vi "Save.vi"() -> ()   [LabVIEW 2018]
uses:
  <vilib>/express/express shared/transition.llb/Dynamic To Waveform Array.vi
  <vilib>/express/express signal manip/GetorSetDDTAttributes/Set DDT Attributes/SetT0.vi
  <vilib>/express/express shared/transition.llb/Waveform Array To Dynamic.vi
  <vilib>/express/express signal manip/GetorSetDDTAttributes/Set DDT Attributes/Set DDT Properties.xnode
panel:
  in  "Stop":bool
  in  "Array":dbl[](array[numeric])
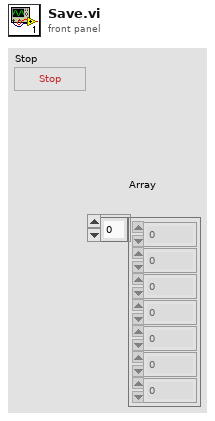
[diagram p1: front panel]
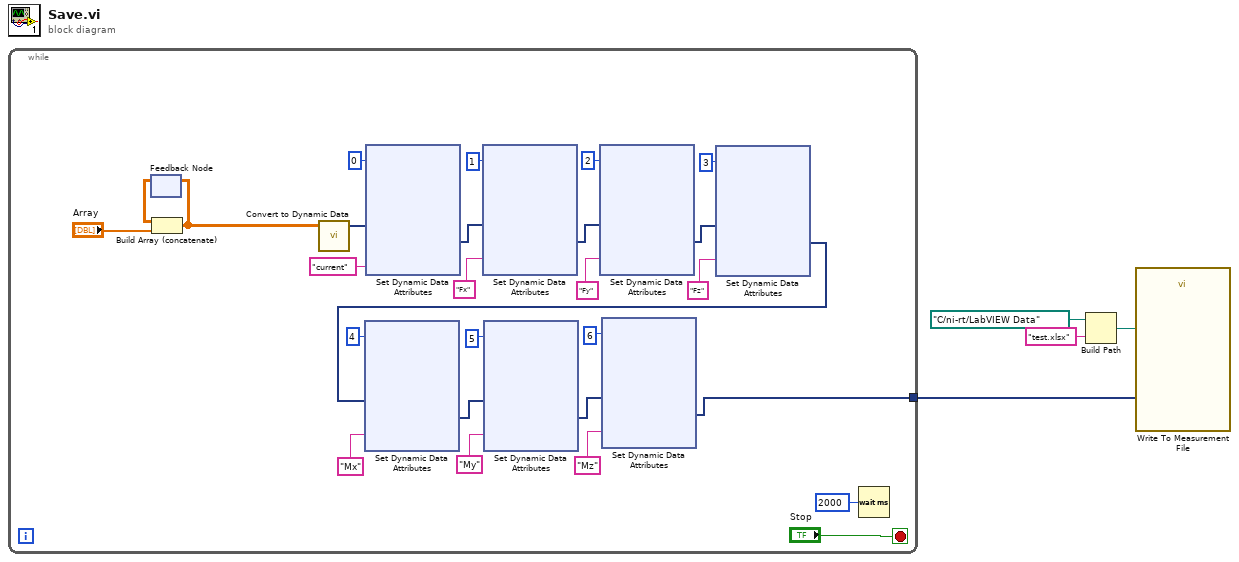
[diagram p0: block diagram]
diagram:
  n1 = while {
    tunnel: [w7] -> w1
    stop <- "Stop" stop-if-true
    n2 = feedback #1() -> (w10:dbl[][])  [unwired: 1 in]
    n3 = Build Array (concatenate)(w10, "Array") -> (w5:dbl[][])
    n4 = feedback-in #1(w5) -> ()
    n5 = call "Convert to Dynamic Data"("2D Array"=w5) -> ("Dynamic Data Type"=w30:dynamicdata)  [unwired: 3 in]
    n6 = xnode "Set Dynamic Data Attributes"("Signals In"=w30, "Signal Name"="current", "Signal Index"=0) -> ("Signals Out"=w28:dynamicdata)  [unwired: 1 in, 1 out]
    n7 = xnode "Set Dynamic Data Attributes"("Signals In"=w28, "Signal Name"="Fx", "Signal Index"=1) -> ("Signals Out"=w23:dynamicdata)  [unwired: 1 in, 1 out]
    n8 = xnode "Set Dynamic Data Attributes"("Signals In"=w23, "Signal Name"="Fy", "Signal Index"=2) -> ("Signals Out"=w14:dynamicdata)  [unwired: 1 in, 1 out]
    n9 = xnode "Set Dynamic Data Attributes"("Signals In"=w14, "Signal Name"="Fz", "Signal Index"=3) -> ("Signals Out"=w18:dynamicdata)  [unwired: 1 in, 1 out]
    n10 = xnode "Set Dynamic Data Attributes"("Signals In"=w18, "Signal Name"="Mx", "Signal Index"=4) -> ("Signals Out"=w15:dynamicdata)  [unwired: 1 in, 1 out]
    n11 = xnode "Set Dynamic Data Attributes"("Signals In"=w15, "Signal Name"="My", "Signal Index"=5) -> ("Signals Out"=w11:dynamicdata)  [unwired: 1 in, 1 out]
    n12 = xnode "Set Dynamic Data Attributes"("Signals In"=w11, "Signal Name"="Mz", "Signal Index"=6) -> ("Signals Out"=w7:dynamicdata)  [unwired: 1 in, 1 out]
    n13 = Wait (ms)(milliseconds to wait=u32 2000) -> ()  [unwired: 1 out]
  }
  n14 = Build Path(base path=path "C:/ni-rt/LabVIEW Data", name or relative path="test.xlsx") -> (appended path=w4:path)
  n15 = call "Write To Measurement File"("Signals"=w1, "Filename"=w4) -> ()  [unwired: 15 in, 3 out]
